vi "Create Secure Profile If Does Not Exist.vi"(7 "Base Profile":string, 8 "error in (no error)":errorcluster, 9 "New Profile Name":string, 11 "Security Settings":T1={"Basic Security Settings"={"Identity Certificate Authority (CA)"=path "", "Identity Certificate (Signed by Identity CA)"=path "", "Private Key"=path "", "Permissions Certificate Authority (CA)"=path "", "Governance Document (Signed by Permissions CA)"=path "", "Permissions Document (Signed by Permissions CA)"=path ""}, "Advanced Security Settings"={"Shared Secret Algorithm"="ecdsa-ecdh", "Encryption Algorithm"="aes-128-gcm", "Certificate Revocation List"=path ""}}) -> (0 "error out":errorcluster, 1 "New Profile Name Output":string)   [LabVIEW 2012]
doc: "Creates a Security configuration if the provided name does not exist."
uses:
  RTI/GIT_HEAD/connextdds/lvdds.1.0/srcLV/lvdds.1.0_package/Types/RTI DDS Security Settings.ctl
  RTI/GIT_HEAD/connextdds/lvdds.1.0/srcLV/lvdds.1.0_package/Types/RTI DDS Basic Security Settings.ctl
  RTI/GIT_HEAD/connextdds/lvdds.1.0/srcLV/lvdds.1.0_package/Types/RTI DDS Advanced Security Settings.ctl
  RTI/GIT_HEAD/connextdds/lvdds.1.0/srcLV/lvdds.1.0_package/Library/LVDDS_library.lvlib
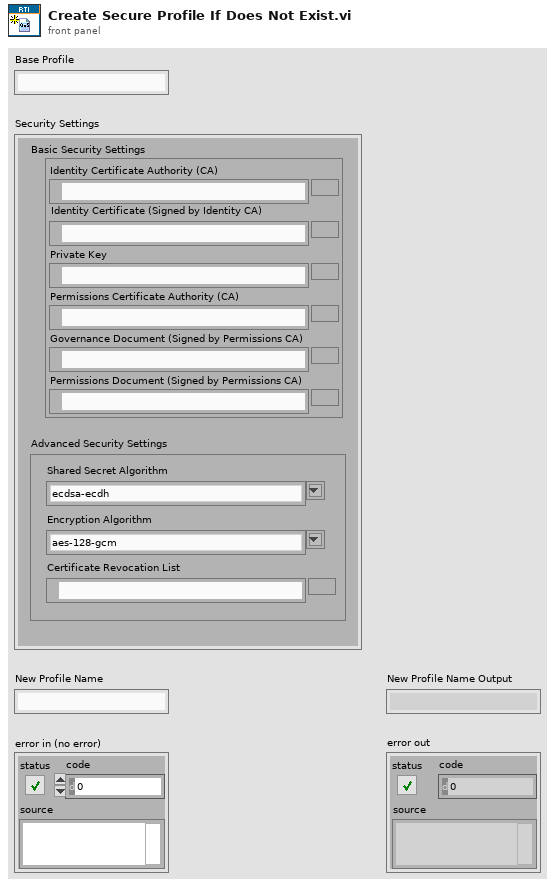
[diagram p1: front panel]
types:
  T1 = typedef "LVDDS_library.lvlib/RTI DDS Security Settings.ctl" = cluster{"Basic Security Settings":T2, "Advanced Security Settings":T3}
  T2 = typedef "LVDDS_library.lvlib/RTI DDS Basic Security Settings.ctl" = cluster{"Identity Certificate Authority (CA)":path, "Identity Certificate (Signed by Identity CA)":path, "Private Key":path, "Permissions Certificate Authority (CA)":path, "Governance Document (Signed by Permissions CA)":path, "Permissions Document (Signed by Permissions CA)":path}
  T3 = typedef "LVDDS_library.lvlib/RTI DDS Advanced Security Settings.ctl" = cluster{"Shared Secret Algorithm":string, "Encryption Algorithm":string, "Certificate Revocation List":path}
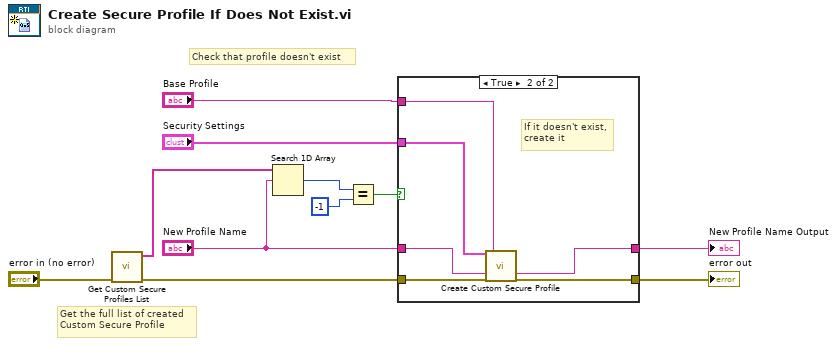
[diagram p0: block diagram]
diagram:
  # "Check that profile doesn't exist"
  # "Get the full list of created \nCustom Secure Profile"
  n1 = call "Get Custom Secure Profiles List.vi"("error in (no error)"="error in (no error)") -> ("error out"=w6:errorcluster, "Array of Customs Secure Profiles"=w8:string[])  [unwired: 9 in]
  n2 = Search 1D Array(1D array=w8, element="New Profile Name") -> (index of element=w10:i32)  [unwired: 1 in]
  n3 = Equal?(x=w10, y=-1 ("x")) -> (x = y?=w11:bool)
  n4 = case shown="True" w11 {
    tunnel: w6 -> [w13 w19]
    tunnel: [w13 w18] -> w5
    tunnel: "New Profile Name" -> [w12 w17]
    tunnel: "Base Profile" -> [_ w14]
    tunnel: "Security Settings" -> [_ w16]
    tunnel: [w12 w15] -> w2
    frame False {
      # "If it already exists, \ndo nothing."
    }
    frame True {
      # "If it doesn't exist,\ncreate it"
      n5 = call "Create Custom Secure Profile.vi"("Security Settings"=w16, "New Custom Secure Profile Name"=w17, "error in (no error)"=w19, "DomainParticipant Base Profile Name"=w14) -> ("Custom Secure Profile Name Output"=w15:string, "error out"=w18:errorcluster)  [unwired: 14 in]
    }
  }
  "error out" <- w5
  "New Profile Name Output" <- w2
